vi "Terminate.vi"(8 "error in (no error)":errorcluster, 10 "Message in":refnum<class "TerminateMessage.lvclass">, 11 "DAQMH121119OrcaFlash in":refnum<class "DAQOrcaFlash.lvclass">) -> (0 "error out":errorcluster, 3 "DAQMH121119OrcaFlash out":refnum<class "DAQOrcaFlash.lvclass">)   [LabVIEW 2012, in "DAQOrcaFlash.lvclass"]
doc: "This member function is called when the statemachine in the run.vi receives an 'terminate' command. It closes the RabbitMQ connection. \n\nOverride this member function in your derived class to release all previously acquired resources (but don't forget to call the parent method). If your component has subcomponents, they count as resources, and you have to release them by calling their own terminate functions."
uses:
  DAQOrcaFlash.lvclass
  <vilib>/Distrio/Murmex/TerminateMessage/TerminateMessage.lvclass
  <vilib>/Distrio/Murmex/StopMessage/StopMessage.lvclass
  DAQOrcaFlash.lvclass/DAQOrcaFlash.ctl
  <vilib>/Distrio/Murmex/Murmex/Murmex.lvclass
panel:
  # "This method is called when the TERMINATE\ntrigger is sent. \n\nOverride this method when your component needs to\nrespond to this trigger. \n\nCall parent for proper implementation"
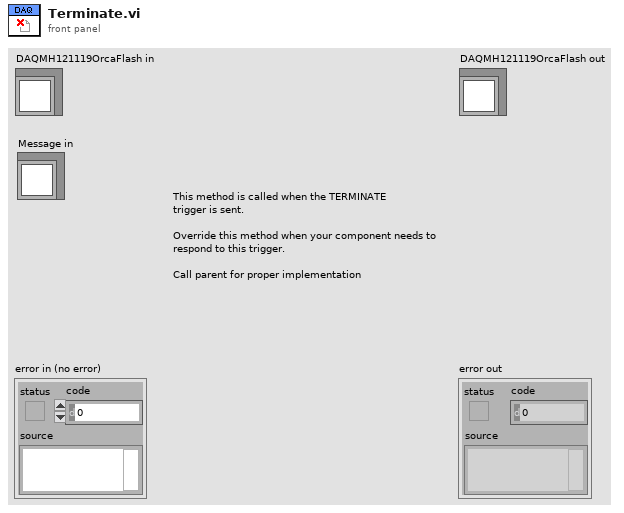
[diagram p1: front panel]
types:
  T1 = typedef "IMAQ Image.ctl" = refnum<image>
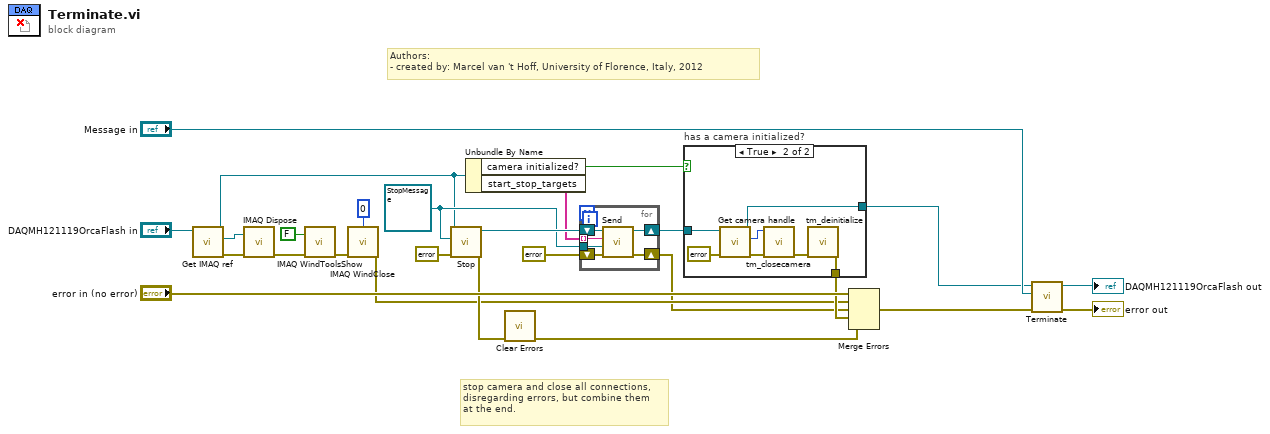
[diagram p0: block diagram]
diagram:
  w8 = refnum<class "StopMessage.lvclass"> refnum ("Message in")
  # "stop camera and close all connections,\ndisregarding errors, but combine them\nat the end."
  # "Authors: \n- created by: Marcel van 't Hoff, University of Florence, Italy, 2012"
  n1 = call "Get IMAQ ref.vi"("DAQMH121119OrcaFlash in"="DAQMH121119OrcaFlash in") -> ("error out"=w18:errorcluster, "IMAQ reference"=w19:T1, "DAQMH121119OrcaFlash out"=w7:refnum<class "DAQOrcaFlash.lvclass">)  [unwired: 8 in]
  n2 = call "IMAQ Dispose"("Image"=w19, "error in (no error)"=w18) -> ("error out"=w17:errorcluster)  [unwired: 4 in]
  n3 = call "IMAQ WindToolsShow"("Hide/Show (Show)"=FALSE, "error in (no error)"=w17) -> ("error out"=w16:errorcluster)  [unwired: 3 in, 1 out]
  n4 = call "IMAQ WindClose"("Window Number (0...15)"=0, "error in (no error)"=w16) -> ("error out"=w14:errorcluster)  [unwired: 4 in]
  n5 = call-dynamic "Stop.vi"("error in (no error)"=errorcluster {"status"=FALSE, "code"=0, "source"=""}, "Message in"=w8, "DAQMH121119OrcaFlash in"=w7) -> ("error out"=w23:errorcluster, "DAQMH121119OrcaFlash out"=w13:refnum<class "DAQOrcaFlash.lvclass">)  [unwired: 7 in]
  n6 = Unbundle By Name(w7) -> ("camera initialized?"=w6:bool, "start_stop_targets"=w10:string[])
  n7 = call <vilib>:"Clear Errors.vi"("error in (no error)"=w23) -> ("error out"=w21:errorcluster)  [unwired: 6 in]
  n8 = for {
    tunnel: w10 -> [w29] mode=indexing
    shift-right: [w31] -> w12
    shift-left: w13 -> [w32]
    shift-right: [w28] -> w9
    shift-left: errorcluster {"status"=FALSE, "code"=0, "source"=""} ("error in (no error)") -> [w30]
    tunnel: w8 -> [w27]
    n9 = call <vilib>:"Send.vi"("error in (no error)"=w30, "Message"=w27, "recipient"=w29, "Murmex in"=w32) -> ("error out"=w28:errorcluster, "Murmex out"=w31:refnum<class "DAQOrcaFlash.lvclass">)  [unwired: 6 in]
  }
  n10 = case "has a camera initialized?" shown="True" w6 {
    tunnel: [w33 w40] -> w2
    tunnel: [_ w35] -> w22
    tunnel: w12 -> [w33 w34]
    frame False {
    }
    frame True {
      n11 = call "Get camera handle.vi"("error in (no error)"=errorcluster {"status"=FALSE, "code"=0, "source"=""}, "DAQMH121119OrcaFlash in"=w34) -> ("error out"=w37:errorcluster, "cam handle"=w38:u32, "DAQMH121119OrcaFlash out"=w40:refnum<class "DAQOrcaFlash.lvclass">)  [unwired: 7 in]
      n12 = call <userlib>:"tm_closecamera.vi"("error in (no error)"=w37, "Handle in"=w38) -> ("error out"=w39:errorcluster)  [unwired: 9 in]
      n13 = call <userlib>:"tm_deinitialize.vi"("error in (no error)"=w39) -> ("error out"=w35:errorcluster)  [unwired: 10 in]
    }
  }
  n14 = Merge Errors("error in (no error)", w14, w9, w22, w21) -> (w1:errorcluster)
  n15 = call-parent "Terminate.vi"("error in (no error)"=w1, "Message in"="Message in", "Murmex in"=w2) -> ("error out"=→"error out":errorcluster, "Murmex out"=→"DAQMH121119OrcaFlash out":refnum<class "DAQOrcaFlash.lvclass">)  [unwired: 7 in]
